vi "Read CSV01.vi"(8 "error in (no error)":errorcluster caption="Error In", 9 "Modules In":T1[](array[typedef]), 10 "Read?":bool, 11 "Data Monitor":path) -> (0 "error out":errorcluster caption="Error Out", 1 "Modules":T1[](array[typedef]))   [LabVIEW 2020]
uses:
  0007 Controls/Data Modules.ctl
  0007 Controls/Data Element Single.ctl
  <vilib>/Utility/miscctls.llb/LVMapReplaceAction.ctl
  <vilib>/Utility/file.llb/Write Delimited Spreadsheet (string).vi
  <vilib>/Utility/file.llb/Read Delimited Spreadsheet (string).vi
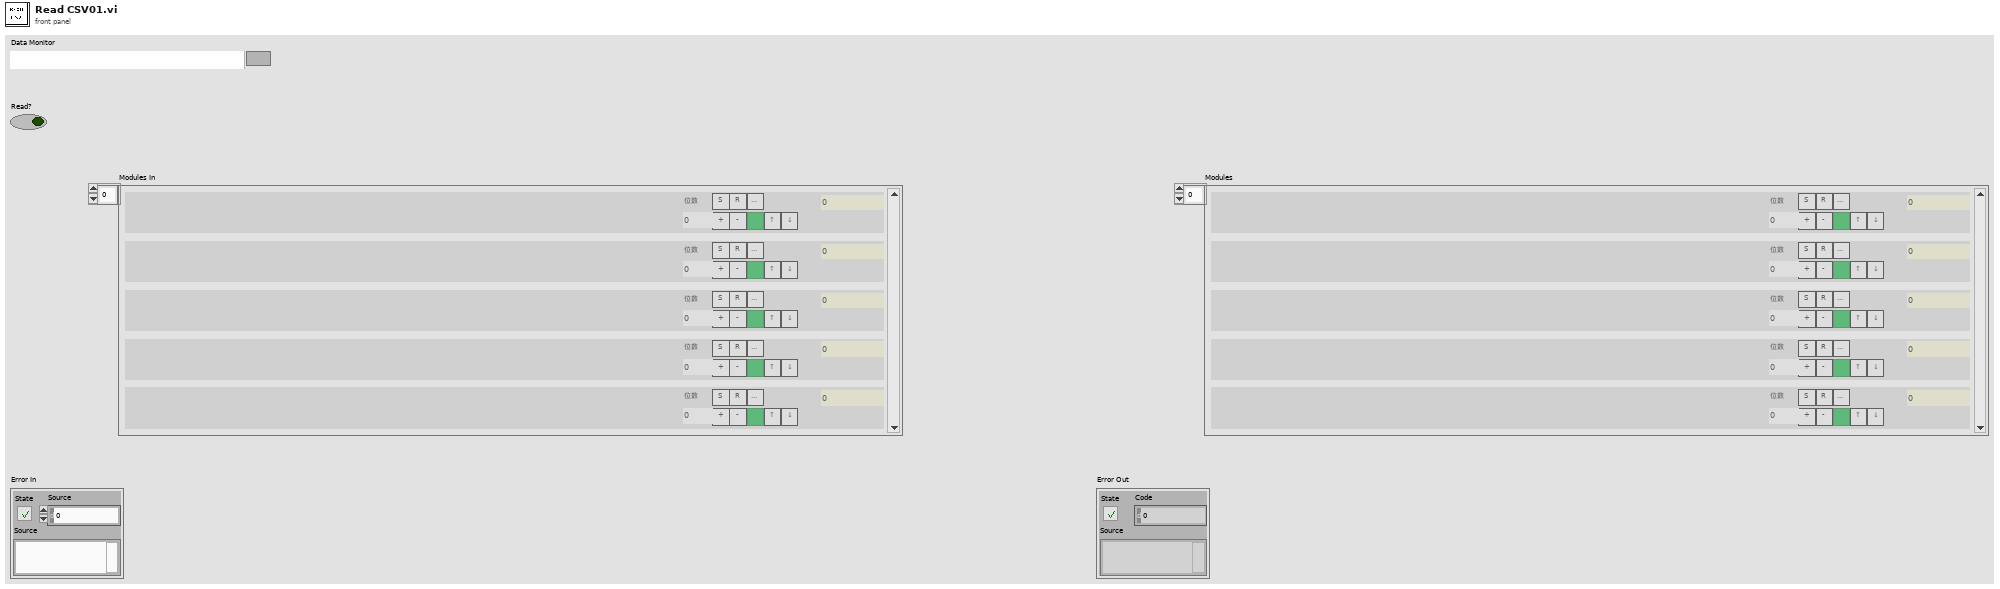
[diagram p1: front panel]
types:
  T1 = typedef "Data Modules.ctl" = cluster{"Names":cluster{"Module Name":string, "Set Value":string, "Real Value":string, "FB Value":string, "Unit":string, "Identifier":string, "IdentifierW":string, "Decimal":string, "AS":bool, "AR":bool, "Con":bool}, "Data":T2[], "Digit":dbl}
  T2 = typedef "Data Element Single.ctl" = cluster{"Name":string, "Set Value":string, "Real Value":string, "FB Value":string, "Unit":string, "Identifier":string, "Write Name":string, "Decimal":u16, "AS":bool, "AR":bool, "ALM":bool, "Up":bool, "Down":bool}
  T3 = typedef "LVMapReplaceAction.ctl" = enum32{"Modify Entry only if found", "Add or Modify Entry", "Delete Entry"}
  T4 = cluster{"Module Name":string, "Set Value":string, "Real Value":string, "FB Value":string, "Unit":string, "Identifier":string, "IdentifierW":string, "Decimal":string, "AS":bool, "AR":bool, "Con":bool}
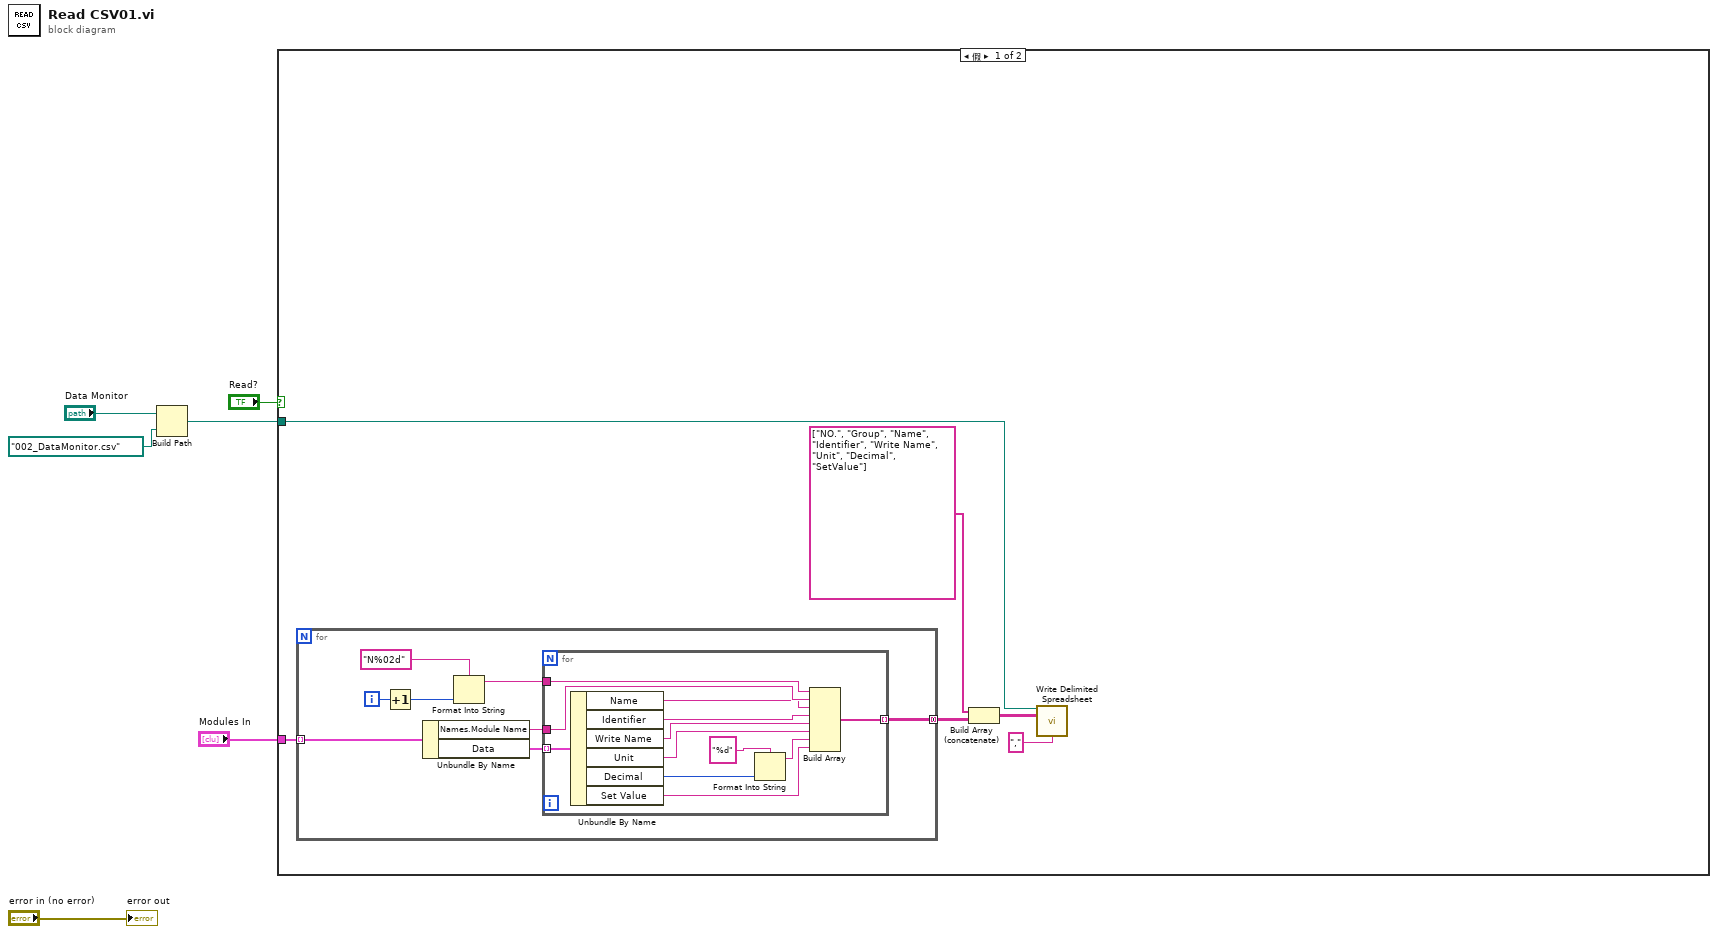
[diagram p0: block diagram]
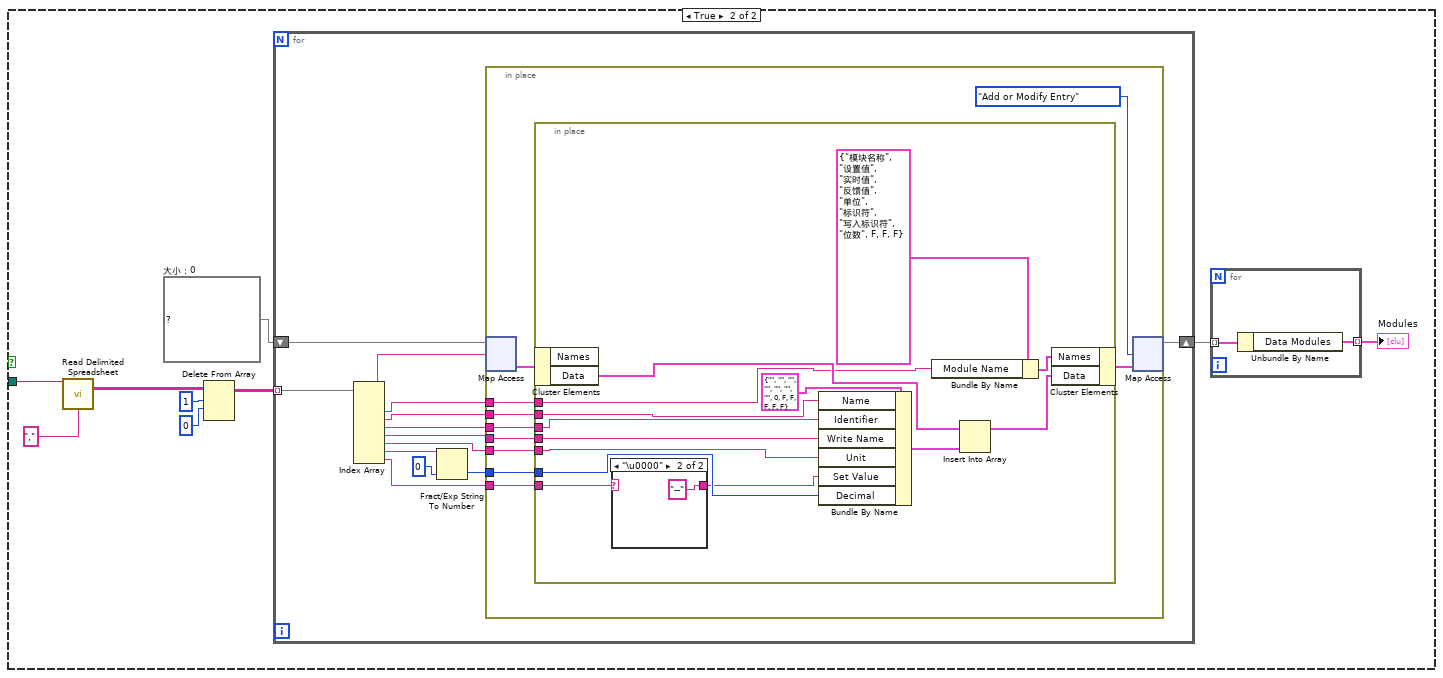
[diagram p2: hidden frame]
diagram:
  n1 = Build Path(base path="Data Monitor", name or relative path=path "002_DataMonitor.csv" ("名称或相对路径")) -> (appended path=w1:path)
  n2 = case shown="假" "Read?" {
    tunnel: w1 -> [w7 w33]
    tunnel: "Modules In" -> [w12 _]
    frame False {
      n3 = for {
        tunnel: w12 -> [w20] mode=indexing
        tunnel: [w17] -> w8 mode=concatenating
        i -> [w16]
        n4 = Increment(x=w16) -> (x+1=w14:i32)
        n5 = Unbundle By Name(w20) -> ("Names.Module Name"=w18:string, "Data"=w19:T2[])
        n6 = Format Into String(format string="N%02d" ("格式字符串"), w14) -> (resulting string=w13:string)  [unwired: 2 in, 1 out]
        n7 = for {
          tunnel: w19 -> [w32] mode=indexing
          tunnel: w18 -> [w31]
          tunnel: [w29] -> w17 mode=indexing
          tunnel: w13 -> [w28]
          n8 = Unbundle By Name(w32) -> ("Name"=w30:string, "Identifier"=w25:string, "Write Name"=w24:string, "Unit"=w23:string, "Decimal"=w26:u16, "Set Value"=w21:string)
          n9 = Format Into String(format string="%d" ("格式字符串"), w26) -> (resulting string=w22:string)  [unwired: 2 in, 1 out]
          n10 = Build Array(w28, w31, w30, w25, w24, w23, w22, w21) -> (w29:string[])
        }
      }
      n11 = Build Array (concatenate)(string[] ["NO.", "Group", "Name", "Identifier", "Write Name", "Unit", "Decimal", "SetValue"], w8) -> (w9:string[][])
      n12 = call-poly <vilib>:"Write Delimited Spreadsheet.vi"("file path (dialog if empty)"=w7, "2D data"=w9, "delimiter (\\t)"="," ("delimiter (\\t)")) -> ()  [unwired: 11 in, 2 out]
    }
    frame True {
      w37 = map{string, T1} {}  # 大小：0
      n13 = call-poly <vilib>:"Read Delimited Spreadsheet.vi"("file path (dialog if empty)"=w33, "delimiter (\\t)"="," ("delimiter (\\t)")) -> ("all rows"=w40:string[][])  [unwired: 8 in, 5 out]
      n14 = Delete From Array(array=w40, length=1 ("长度"), index (row)=0 ("索引 (行)")) -> (array with subset deleted=w36:string[][])  [unwired: 1 in, 1 out]
      n15 = for {
        shift-right: [w53] -> w35
        shift-left: w37 -> [w55]
        tunnel: w36 -> [w56] mode=indexing
        n16 = Index Array(array=w56) -> (element #1=w54:string, element #2=w52:string, element #3=w51:string, element #4=w50:string, element #5=w49:string, element #6=w48:string, element #7=w45:string, element #8=w44:string)  [unwired: 8 in]
        n17 = Fract/Exp String To Number(string=w45, default (0 dbl)=u16 0 ("Decimal")) -> (number=w47:u16)  [unwired: 2 in, 1 out]
        n18 = in-place {
          in-place-border: w52 -> [w64]
          in-place-border: w51 -> [w62]
          in-place-border: w50 -> [w61]
          in-place-border: w49 -> [w60]
          in-place-border: w48 -> [w59]
          in-place-border: w47 -> [w58]
          in-place-border: w44 -> [w57]
          n19 = in-place-map #1(w55, w54) -> (w65:T1)  [unwired: 1 in, 1 out]
          n20 = in-place {
            in-place-border: w64 -> [w71]
            in-place-border: w62 -> [w76]
            in-place-border: w61 -> [w75]
            in-place-border: w60 -> [w74]
            in-place-border: w59 -> [w73]
            in-place-border: w58 -> [w72]
            in-place-border: w57 -> [w68]
            n21 = in-place-cluster #2(w65) -> ("Data"=w80:T2[])  [unwired: 1 out]
            n22 = case shown="\"\"" w68 {
              selector: w68 -> [w81 _]
              tunnel: [w81 "--"] -> w67
              frame Default {
              }
              frame "\u0000" {
              }
            }
            n23 = Bundle By Name(cluster=T2 {"Name"="", "Set Value"="", "Real Value"="", "FB Value"="", "Unit"="", "Identifier"="", "Write Name"="", "Decimal"=0, "AS"=FALSE, "AR"=FALSE, "ALM"=FALSE, "Up"=FALSE, "Down"=FALSE} ("新元素/子数组"), "Name"=w76, "Identifier"=w75, "Write Name"=w74, "Unit"=w73, "Set Value"=w67, "Decimal"=w72) -> (w77:T2)
            n24 = Bundle By Name(cluster=T4 {"Module Name"="模块名称", "Set Value"="设置值", "Real Value"="实时值", "FB Value"="反馈值", "Unit"="单位", "Identifier"="标识符", "IdentifierW"="写入标识符", "Decimal"="位数", "AS"=FALSE, "AR"=FALSE, "Con"=FALSE} ("Names"), "Module Name"=w71) -> (w69:T4)
            n25 = Insert Into Array(array=w80, new element=w77) -> (w79:T2[])  [unwired: 1 in]
            n26 = in-place-cluster #2("Names"=w69, "Data"=w79) -> (w63:T1)
          }
          n27 = in-place-map #1(w63, LVMapReplaceAction."Add or Modify Entry" ("操作")) -> (w53:map{string, T1})  [unwired: 2 out]
        }
      }
      n28 = for {
        tunnel: w35 -> [w43] mode=indexing
        tunnel: [w42] -> w34 mode=indexing
        n29 = Unbundle By Name(w43) -> ("Data Modules"=w42:T1)
      }
      "Modules" <- w34
    }
  }
  "error out" <- "error in (no error)"
